vi "Slider_Module.vi"(7 "Slider":dbl(slide) scale=0.0..10.0, 11 "Error_In":errorcluster) -> (15 "Error_Out":errorcluster)   [LabVIEW 2023]
doc: "This is the main module to generate the data ( Recording the data )"
uses:
  Controls/Operation.ctl
  Controls/Event_Data_and_Parameter.ctl
  Controls/Event_Data.ctl
  LV2/UE_C_LV2.vi
panel:
  out "Record_State":string
  in  "PlayBack?":bool
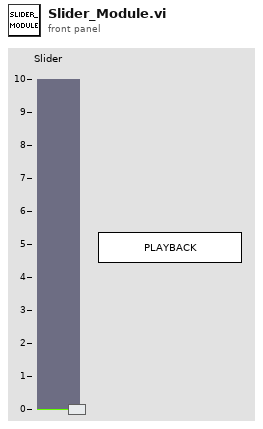
[diagram p1: front panel]
types:
  T1 = typedef "Event_Data.ctl" = cluster{"Event_Data":dbl, "PlayBack?":bool}
  T2 = typedef "Event_Data_and_Parameter.ctl" = cluster{"Event_Data":dbl[], "Generate_Event":bool, "Playback?":bool, "Index":i32}
  T3 = typedef "Operation.ctl" = enum16{"Create_UE", "Generate_UE", "Destroy_UE", "Get_UE_Reference"}
  T4 = enum32{"Bad", "Idle", "Run top level", "Running"}
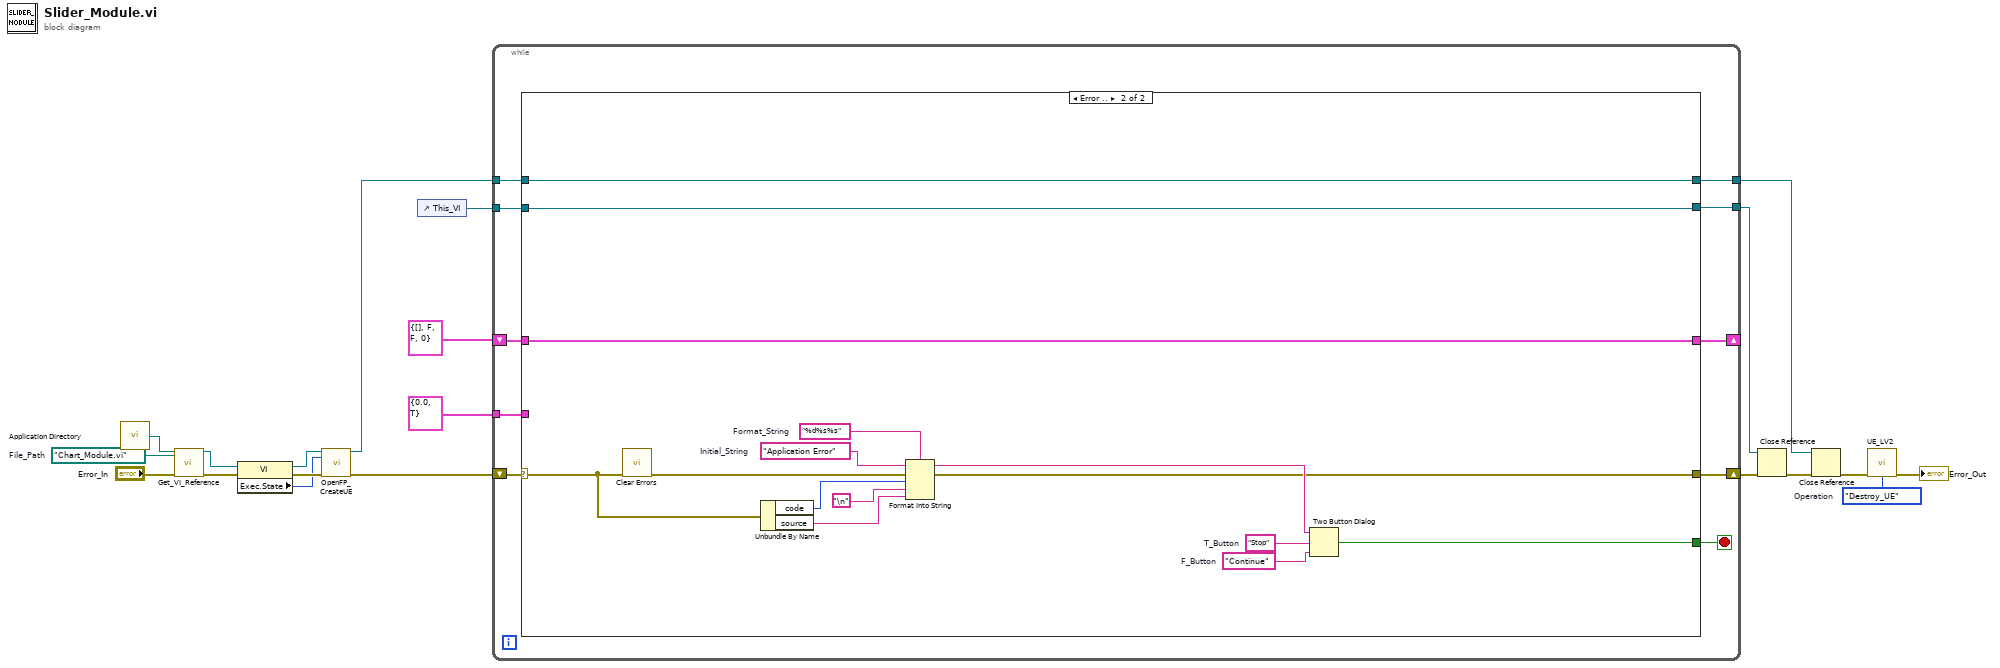
[diagram p0: block diagram]
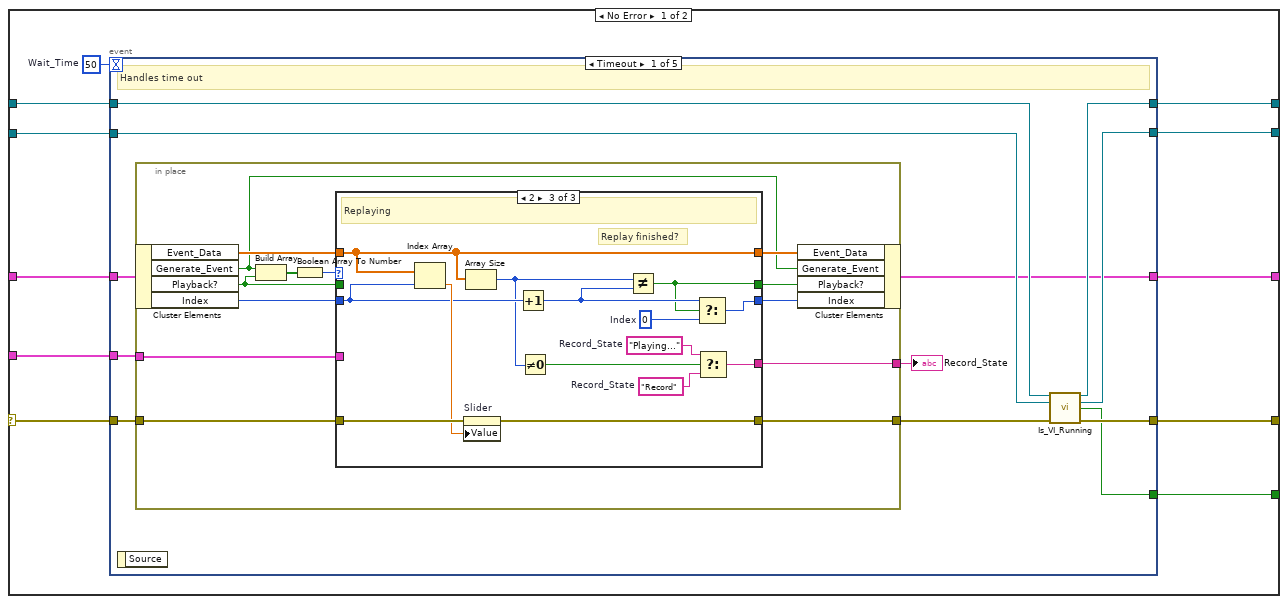
[diagram p2: hidden frame]
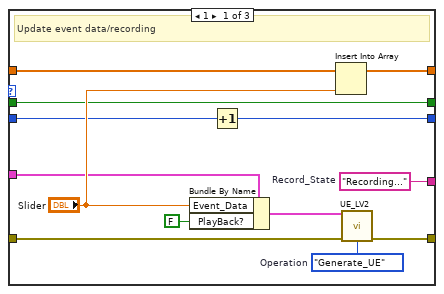
[diagram p3: hidden frame]
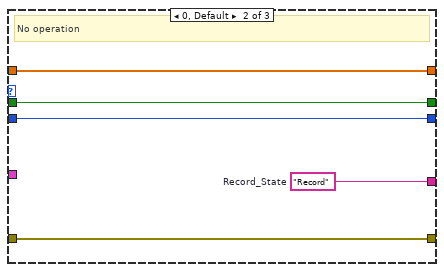
[diagram p4: hidden frame]
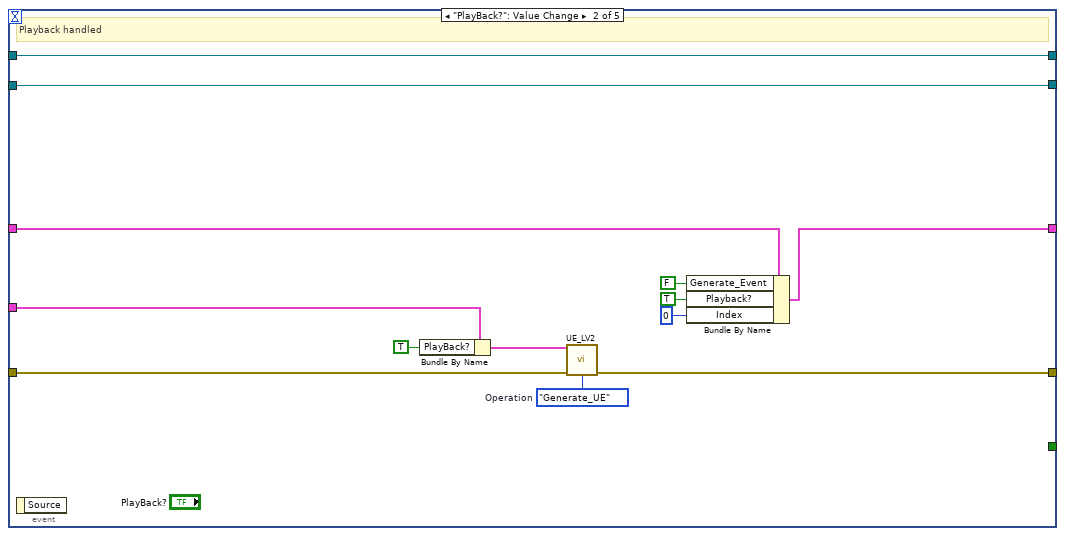
[diagram p5: hidden frame]
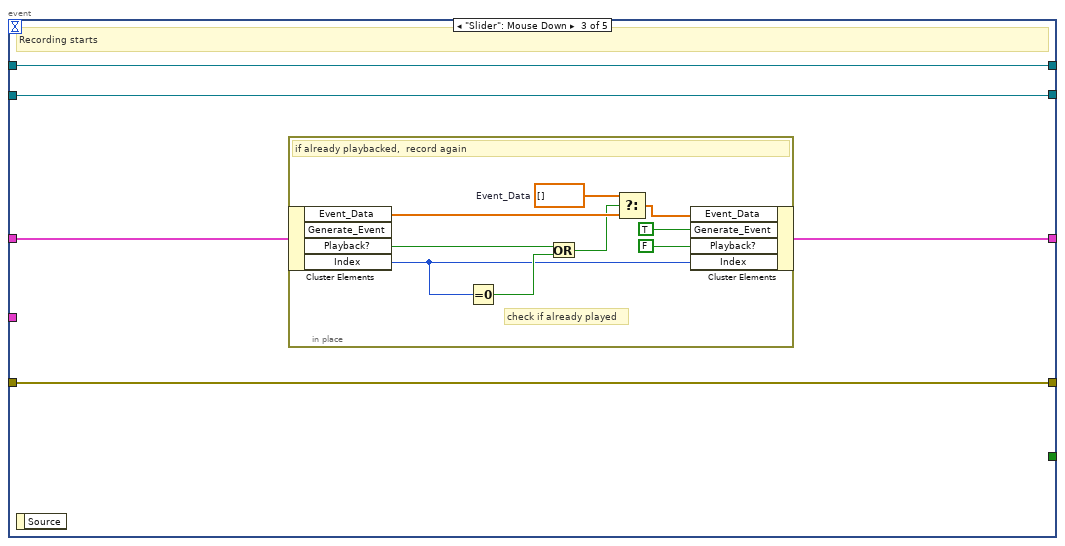
[diagram p6: hidden frame]
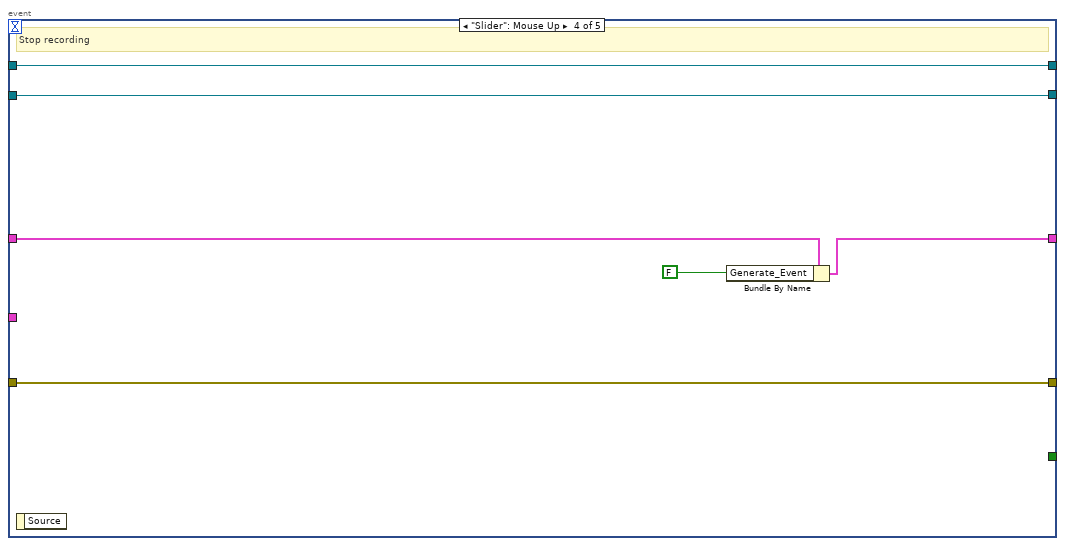
[diagram p7: hidden frame]
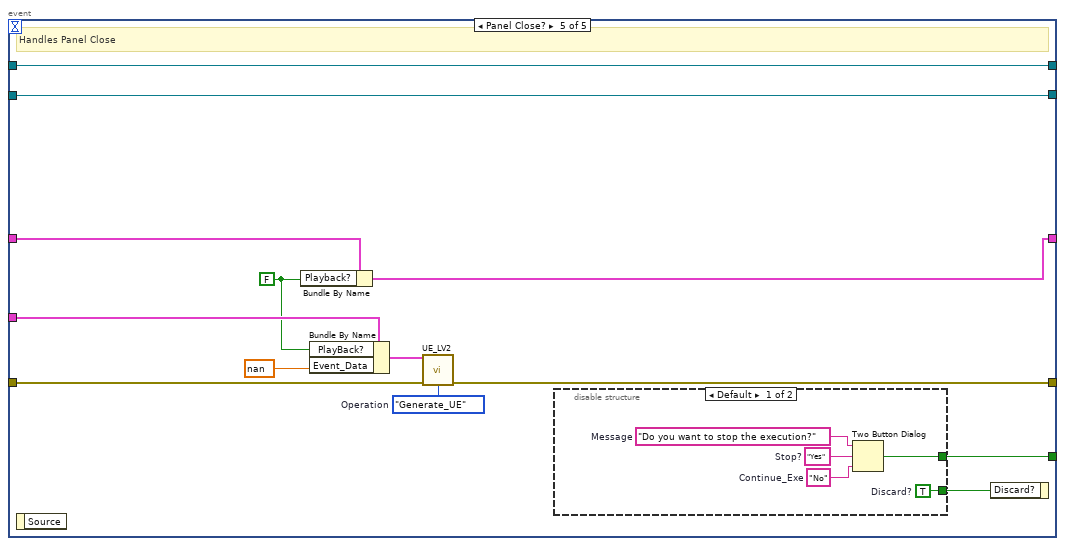
[diagram p8: hidden frame]
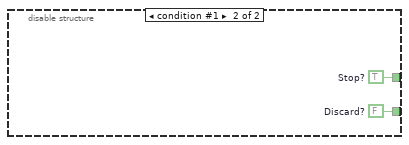
[diagram p9: hidden frame]
diagram:
  w13 = Operation."Destroy_UE"  # Operation
  w17 = path "Chart_Module.vi"  # File_Path
  n1 = call <vilib>:"Application Directory.vi"() -> ("Application Directory"=w18:path)
  n2 = call "Get_VI_Reference.vi"("Application_Directory"=w18, "File_Path"=w17, "Error_In"="Error_In") -> ("VI_Reference"=w16:refnum<vi>, "Error_Out"=w19:errorcluster)  [unwired: 11 in]
  n3 = property on="Property Node" class="VI"(reference=w16, error in=w19) -> (reference out=w5:refnum<vi>, error out=w6:errorcluster, "Exec.State"=w4:T4)
  n4 = call "OpenFP_CreateUE.vi"("VI_Reference_In"=w5, "Exec.State"=w4, "Error_In"=w6) -> ("VI_Reference_Out"=w3:refnum<vi>, "Error_Out"=w2:errorcluster)  [unwired: 11 in]
  n5 = control-ref of="This_VI"() -> (w12:refnum<vi>)
  n6 = while {
    shift-right: [w27] -> _
    shift-left: T2 {"Event_Data"=[], "Generate_Event"=FALSE, "Playback?"=FALSE, "Index"=0} -> [w26]
    tunnel: w3 -> [w25]
    tunnel: w12 -> [w24]
    tunnel: [w23] -> w11
    tunnel: [w22] -> w8
    tunnel: T1 {"Event_Data"=0.0, "PlayBack?"=TRUE} ("Event_Data") -> [w21]
    shift-right: [w29] -> w15
    shift-left: w2 -> [w30]
    stop <- w28 stop-if-true
    n7 = case shown="Error .." w30 {
      selector: w30 -> [w40 w158]
      tunnel: [w41 w159] -> w29
      tunnel: [w38 w155] -> w28
      tunnel: [w32 w154] -> w27
      tunnel: w26 -> [w37 w154]
      tunnel: w25 -> [w36 w153]
      tunnel: w24 -> [w35 w152]
      tunnel: [w34 w152] -> w23
      tunnel: [w33 w153] -> w22
      tunnel: w21 -> [w31 _]
      frame No Error {
        w39 = 50  # Wait_Time
        n8 = event shown="[0] Timeout" {
          selector: _ -> [_ _ _ _ _]
          dyn-events: _ -> [_ _ _ _ _]
          timeout: w39 -> [_ _ _ _ _]
          tunnel: [w51 w110 w116 w130 w136] -> w41
          tunnel: w40 -> [w53 w111 w116 w130 w142]
          tunnel: [w46 _ _ _ w133] -> w38
          tunnel: w37 -> [w45 w106 w113 w131 w139]
          tunnel: w36 -> [w50 w100 w115 w127 w143]
          tunnel: w35 -> [w49 w101 w114 w126 w144]
          tunnel: [w48 w101 w114 w126 w144] -> w34
          tunnel: [w47 w100 w115 w127 w143] -> w33
          tunnel: [w44 w105 w112 w129 w138] -> w32
          tunnel: w31 -> [w42 w99 _ _ w137]
          event Timeout {
            # "Handles time out"
            n9 = event-data() -> ()  [unwired: 1 in, 1 out]
            n10 = in-place "In Place Element Structure" {
              in-place-border: w53 -> [w66]
              in-place-border: [w63] -> w52
              in-place-border: [w58] -> w43
              in-place-border: w42 -> [w57]
              n11 = in-place-cluster #1(w45) -> ("Event_Data"=w62:dbl[], "Generate_Event"=w59:bool, "Playback?"=w55:bool, "Index"=w54:i32)
              n12 = Build Array(w59, w55) -> (w65:bool[])
              n13 = Boolean Array To Number(Boolean array=w65) -> (number=w64:u32)
              n14 = case shown="2" w64 {
                tunnel: w66 -> [w79 w82 w98]
                tunnel: [w78 w82 w97] -> w63
                tunnel: [w76 w84 w95] -> w61
                tunnel: w62 -> [w75 w84 w95]
                tunnel: [w67 w83 w94] -> w60
                tunnel: w54 -> [w68 w83 w88]
                tunnel: [w71 w80 w90] -> w58
                tunnel: w57 -> [w70 _ _]
                tunnel: [w69 w81 w87] -> w56
                tunnel: w55 -> [w69 w81 _]
                frame 1 {
                  w71 = "Recording..."  # Record_State
                  w77 = Operation."Generate_UE"  # Operation
                  # "Update event data/recording"
                  n15 = Bundle By Name(cluster=w70, "Event_Data"="Slider", "PlayBack?"=FALSE) -> (w73:T1)
                  n16 = Increment(x=w68) -> (x+1=w67:i32)
                  n17 = Insert Into Array(array=w75, new element="Slider") -> (w76:dbl[])  [unwired: 1 in]
                  n18 = call-poly "UE_LV2.vi"("Event_Data"=w73, "Error_In"=w79, "Operation"=w77) -> ("Error_Out"=w78:errorcluster)  [unwired: 11 in, 1 out]
                }
                frame 0, Default {
                  w80 = "Record"  # Record_State
                  # "No operation"
                }
                frame 2 {
                  w89 = "Record"  # Record_State
                  w93 = 0  # Index
                  w91 = "Playing..."  # Record_State
                  # "Replay finished?"
                  # "Replaying"
                  n19 = Index Array(array=w95, index=w88) -> (element=w96:dbl)
                  n20 = property on="Slider" class="Slide (strict)"(error in=w98, "Value"=w96) -> (error out=w97:errorcluster)  [unwired: 1 in, 1 out]
                  n21 = Array Size(array=w95) -> (size(s)=w86:i32)
                  n22 = Increment(x=w88) -> (x+1=w92:i32)
                  n23 = Not Equal To 0?(x=w86) -> (x != 0?=w85:bool)
                  n24 = Not Equal?(x=w86, y=w92) -> (x != y?=w87:bool)
                  n25 = Select(t=w92, s=w87, f=w93) -> (s? t:f=w94:i32)
                  n26 = Select(t=w91, s=w85, f=w89) -> (s? t:f=w90:string)
                }
              }
              n27 = in-place-cluster #1("Event_Data"=w61, "Generate_Event"=w59, "Playback?"=w56, "Index"=w60) -> (w44:T2)
            }
            "Record_State" <- w43
            n28 = call "Is_VI_Running.vi"("Other_VI_Reference_In"=w50, "This_VI_Reference_In"=w49, "Error_In"=w52) -> ("Other_VI_Reference_Out"=w47:refnum<vi>, "This_VI_Reference_Out"=w48:refnum<vi>, "Stop"=w46:bool, "Error_Out"=w51:errorcluster)  [unwired: 9 in]
          }
          event "PlayBack?": Value Change {
            w109 = Operation."Generate_UE"  # Operation
            # "Playback handled"
            n29 = event-data() -> ()  [unwired: 1 in, 1 out]
            n30 = Bundle By Name(cluster=w99, "PlayBack?"=TRUE) -> (w108:T1)
            n31 = call-poly "UE_LV2.vi"("Event_Data"=w108, "Error_In"=w111, "Operation"=w109) -> ("Error_Out"=w110:errorcluster)  [unwired: 11 in, 1 out]
            n32 = Bundle By Name(cluster=w106, "Generate_Event"=FALSE, "Playback?"=TRUE, "Index"=0) -> (w105:T2)
          }
          event "Slider": Mouse Down {
            # "Recording starts"
            n33 = event-data() -> ()  [unwired: 1 in, 1 out]
            n34 = in-place "In Place Element Structure" {
              w122 = dbl[] []  # Event_Data
              # "check if already played"
              # "if already playbacked,  record again"
              n35 = in-place-cluster #2(w113) -> ("Event_Data"=w121:dbl[], "Playback?"=w117:bool, "Index"=w119:i32)  [unwired: 1 out]
              n36 = Equal To 0?(x=w119) -> (x = 0?=w120:bool)
              n37 = Or(x=w117, y=w120) -> (x .or. y?=w118:bool)
              n38 = Select(t=w122, s=w118, f=w121) -> (s? t:f=w123:dbl[])
              n39 = in-place-cluster #2("Event_Data"=w123, "Generate_Event"=TRUE, "Playback?"=FALSE, "Index"=w119) -> (w112:T2)
            }
          }
          event "Slider": Mouse Up {
            # "Stop recording"
            n40 = event-data() -> ()  [unwired: 1 in, 1 out]
            n41 = Bundle By Name(cluster=w131, "Generate_Event"=FALSE) -> (w129:T2)
          }
          event Panel Close? {
            w134 = FALSE
            w141 = Operation."Generate_UE"  # Operation
            # "Handles Panel Close"
            n42 = event-data() -> ()  [unwired: 1 in, 1 out]
            n43 = Bundle By Name(cluster=w139, "Playback?"=w134) -> (w138:T2)
            n44 = Bundle By Name(cluster=w137, "PlayBack?"=w134, "Event_Data"=nan) -> (w140:T1)
            n45 = call-poly "UE_LV2.vi"("Event_Data"=w140, "Error_In"=w142, "Operation"=w141) -> ("Error_Out"=w136:errorcluster)  [unwired: 11 in, 1 out]
            n46 = disable-structure shown="Default" {
              disable-tunnel: [w146 w151] -> w133
              disable-tunnel: [w145 w150] -> w132
              frame condition #0 (active) {
                w145 = TRUE  # Discard?
                w147 = "No"  # Continue_Exe
                w148 = "Yes"  # Stop?
                w149 = "Do you want to stop the execution?"  # Message
                n47 = Two Button Dialog(message=w149, 1:w147, 2:w148) -> (T button?=w146:bool)
              }
              frame condition #1 {
                w150 = FALSE  # Discard?
                w151 = TRUE  # Stop?
              }
            }
            n48 = event-data ("Event Filter Node")("Discard?"=w132) -> ()  [unwired: 1 in, 1 out]
          }
        }
      }
      frame Error {
        w162 = "%d%s%s"  # Format_String
        w163 = "Application Error"  # Initial_String
        w164 = "Stop"  # T_Button
        w165 = "Continue"  # F_Button
        n49 = call <vilib>:"Clear Errors.vi"("error in (no error)"=w158) -> ("error out"=w160:errorcluster)  [unwired: 5 in, 1 out]
        n50 = Unbundle By Name(w158) -> ("code"=w157:i32, "source"=w156:string)
        n51 = Format Into String(format string=w162, initial string=w163, error in=w160, w157, "\n" ("Line Feed Constant"), w156) -> (resulting string=w166:string, error out=w159:errorcluster)
        n52 = Two Button Dialog(message=w166, 1:w165, 2:w164) -> (T button?=w155:bool)
      }
    }
  }
  n53 = Close Reference(reference=w11, error in (no error)=w15) -> (error out=w10:errorcluster)
  n54 = Close Reference(reference=w8, error in (no error)=w10) -> (error out=w9:errorcluster)
  n55 = call-poly "UE_LV2.vi"("Error_In"=w9, "Operation"=w13) -> ("Error_Out"=→"Error_Out":errorcluster)  [unwired: 12 in, 1 out]
